vi "DataStream_RT_Flush Streams.vi"(8 "Error":errorcluster, 11 "Stream Writer Ref":T1) -> (0 "Error Out":errorcluster, 3 "Stream Writer Ref Out":T1)   [LabVIEW 2020]
uses:
  TypeDefs/Cluster_DataStream_RT Writer Refs.ctl
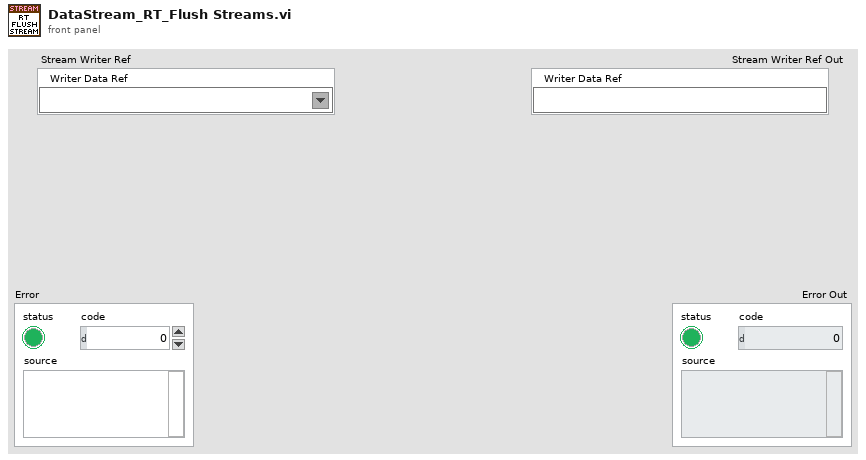
[diagram p1: front panel]
types:
  T1 = typedef "Cluster_DataStream_RT Writer Refs.ctl" = cluster{"Writer Data Ref":refnum<k21>}
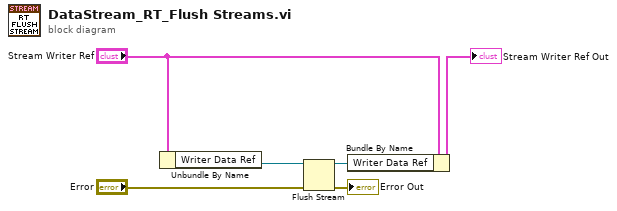
[diagram p0: block diagram]
diagram:
  n1 = Unbundle By Name("Stream Writer Ref") -> ("Writer Data Ref"=w6:refnum<k21>)
  n2 = Flush Stream(8:"Error", 11:w6) -> (0:→"Error Out":errorcluster, 3:w3:refnum<k21>)  [unwired: 2 in, 1 out]
  n3 = Bundle By Name(cluster="Stream Writer Ref", "Writer Data Ref"=w3) -> (→"Stream Writer Ref Out":T1)
